vi "IO.vi"() -> ()   [LabVIEW 2010]
panel:
  out "FPGAVersion":i32
  out "HardwareVersion":i32
  out "FirmwareVersion":string
  out "Digital Output 2":bool[](array[boolean])
  out "Digital Output 1":bool[](array[boolean])
  out "Digital Output 0":bool[](array[boolean])
  out "Digital Input 2":bool[](array[boolean])
  out "Digital Input 1":bool[](array[boolean])
  out "Digital Input 0":bool[](array[boolean])
  out "Analog Output 1":dbl
  out "Analog Output 0":dbl
  out "Analog Input 1":dbl
  out "Analog Input 0":dbl
  in  "Analog Output 1 (set)":dbl=-3.25
  in  "Analog Output 0 (set)":dbl=7.0
  in  "Digital Output 2 (set)":i32=255 format="%02x"
  in  "Digital Output 1 (set)":i32=122 format="%02x"
  in  "Digital Output 0 (set)":i32=3 format="%01x"
  in  "Axis Name":string="X"
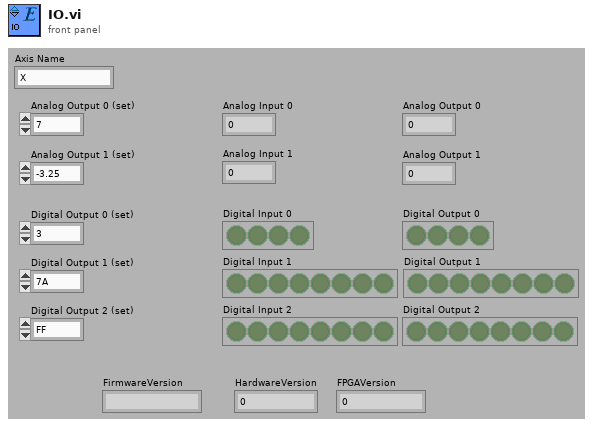
[diagram p1: front panel]
types:
  T1 = typedef "ControllerDiagPacket.ctl" = cluster{"Count":i32, "Packet Time":i64, "Axes":T2[], "error":errorcluster}
  T2 = typedef "AxisDiagPacket.ctl" = cluster{"Axis Name":string, "Acceleration Command":dbl, "Amplifier Temperature":sgl, "Analog Input 0":dbl, "Analog Input 1":dbl, "Analog Output 0":dbl, "Analog Output 1":dbl, "Axis Fault (num)":i32, "Axis Fault (str)":string, "Axis Fault (bits)":cluster{"AmplifierFault":bool, "AmplifierTemperatureFault":bool, "CcwEndOfTravelLimitFault":bool, "CcwSoftwareLimitFault":bool, "CommunicationLostFault":bool, "CwEndOfTravelLimitFault":bool, "CwSoftwareLimitFault":bool, "EmergencyStopFault":bool, "EncoderFault":bool, "ExternalFault":bool, "FeedbackScalingFault":bool, "HallSensorFault":bool, "MarkerSearchFault":bool, "MaxVelocityCommandFault":bool, "MotorTemperatureFault":bool, "None":bool, "OverCurrentFault":bool, "PositionErrorFault":bool, "PositionFeedbackFault":bool, "PowerSupplyFault":bool, "VelocityErrorFault":bool, "VelocityFeedbackFault":bool, "VoltageClampFault":bool}, "Axis Status (num)":i32, "Axis Status (str)":string, "Axis Status (bits)":cluster{"AccelerationPhase":bool, "AutofocusActive":bool, "BrakeOutput":bool, "CalibrationActive":bool, "CalibrationEnabled":bool, "CcwEndOfTravelLimitInput":bool, "CommandShapingFilterDone":bool, "CosineEncoderError":bool, "CurrentClamp":bool, "CwEndOfTravelLimitInput":bool, "DecelerationPhase":bool, "EmergencyStopInput":bool, "Enabled":bool, "GantryMasterActive":bool, "GantryModeActive":bool, "HallAInput":bool, "HallBInput":bool, "HallCInput":bool, "Homed":bool, "HomeLimitInput":bool, "Homing":bool, "InPosition":bool, "InPosition2":bool, "JoystickControl":bool, "MarkerInput":bool, "MasterMotionSuppressed":bool, "MasterSlaveControl":bool, "MotionIsCw":bool, "MoveActive":bool, "None":bool, "PositionCaptureActive":bool, "ServoControl":bool, "SineEncoderError":bool}, "Current Command":sgl, "Current Error":sgl, "Current Feedback":sgl, "Digital Input 0":i32, "Digital Input 1":i32, "Digital Input 2":i32, "Digital Output 0":i32, "Digital Output 1":i32, "Digital Output 2":i32, "Position Feedback Auxiliary":dbl, "Position Command":dbl, "Position Error":dbl, "Position Feedback":dbl, "Program Position Command":dbl, "Program Position Error":dbl, "Program Position Feedback":dbl, "Velocity Command":dbl, "Velocity Error":dbl, "Velocity Feedback":dbl}
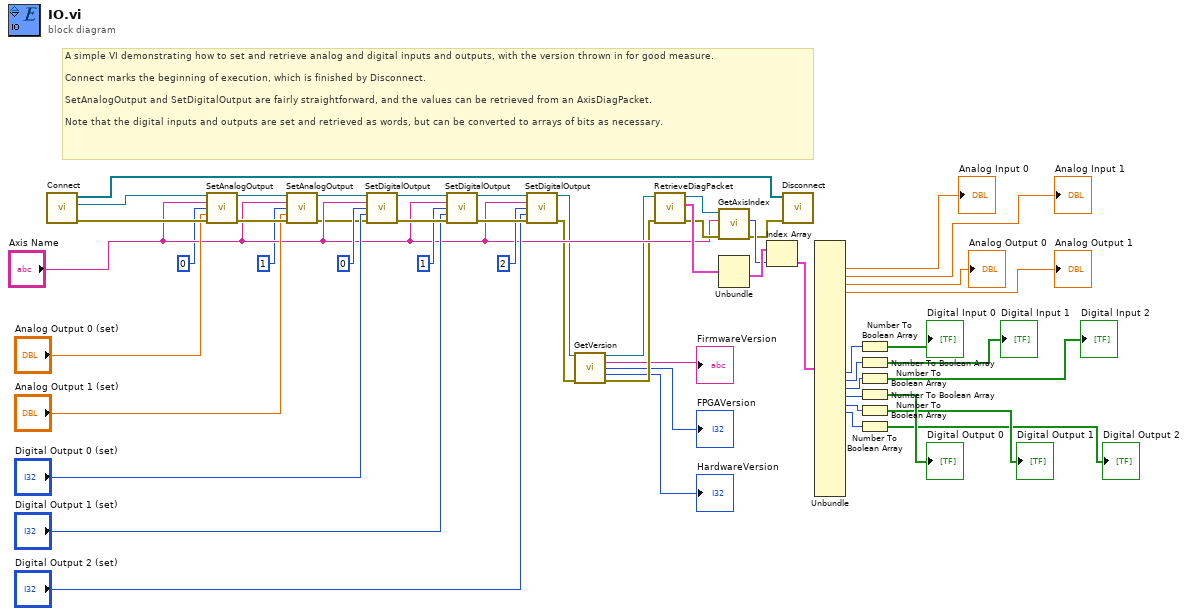
[diagram p0: block diagram]
diagram:
  # "A simple VI demonstrating how to set and retrieve analog and digital inputs and outputs, with the version thrown in for good measure.\n\nConnect marks the beginning of execution, which is finished by Disconnect.\n\nSetAnalogOutput and SetDigitalOutput are fairly straightforward, and the values can be retrieved from an AxisDiagPacket.\n\nNote that the digital inputs and outputs are set and retrieved as words, but can be converted to arrays of bits as necessary."
  n1 = call "Connect.vi"() -> ("error out"=w24:errorcluster, "controller"=w25:refnum<k24>, "controllers"=w7:refnum<k24>[])  [unwired: 9 in]
  n2 = call "SetAnalogOutput.vi"("controller in"=w25, "axis name"="Axis Name", "port"=0 ("Port"), "value"="Analog Output 0 (set)", "error in (no error)"=w24) -> ("controller out"=w23:refnum<k24>, "error out"=w22:errorcluster)  [unwired: 9 in]
  n3 = call "SetAnalogOutput.vi"("controller in"=w23, "axis name"="Axis Name", "port"=1 ("Port"), "value"="Analog Output 1 (set)", "error in (no error)"=w22) -> ("controller out"=w16:refnum<k24>, "error out"=w15:errorcluster)  [unwired: 9 in]
  n4 = call "SetDigitalOutput.vi"("controller in"=w16, "axis name"="Axis Name", "port"=0 ("Port"), "value"="Digital Output 0 (set)", "error in (no error)"=w15) -> ("controller out"=w35:refnum<k24>, "error out"=w33:errorcluster)  [unwired: 9 in]
  n5 = call "SetDigitalOutput.vi"("controller in"=w35, "axis name"="Axis Name", "port"=1 ("Port"), "value"="Digital Output 1 (set)", "error in (no error)"=w33) -> ("controller out"=w34:refnum<k24>, "error out"=w32:errorcluster)  [unwired: 9 in]
  n6 = call "SetDigitalOutput.vi"("controller in"=w34, "axis name"="Axis Name", "port"=2 ("Port"), "value"="Digital Output 2 (set)", "error in (no error)"=w32) -> ("controller out"=w14:refnum<k24>, "error out"=w11:errorcluster)  [unwired: 9 in]
  n7 = call "GetVersion.vi"("controller in"=w14, "error in (no error)"=w11) -> ("controller out"=w13:refnum<k24>, "firmware version"=→"FirmwareVersion":string, "fpga version"=→"FPGAVersion":i32, "hardware version"=→"HardwareVersion":i32, "error out"=w12:errorcluster)  [unwired: 9 in]
  n8 = call "RetrieveDiagPacket.vi"("error in (no error)"=w12, "Controller In"=w13) -> ("error out"=w51:errorcluster, "ControllerDiagPacket"=w52:T1, "Controller Out"=w50:refnum<k24>)  [unwired: 7 in]
  n9 = call "GetAxisIndex.vi"("error in (no error)"=w51, "axis name"="Axis Name", "controller in"=w50) -> ("error out"=w36:errorcluster, "axis index"=w48:i32)  [unwired: 6 in, 1 out]
  n10 = Unbundle(w52) -> ("Axes"=w49:T2[])  [unwired: 3 out]
  n11 = Index Array(array=w49, index=w48) -> (element=w47:T2)
  n12 = call "Disconnect.vi"("error in (no error)"=w36, "controllers"=w7) -> ()  [unwired: 9 in, 1 out]
  n13 = Unbundle(w47) -> ("Analog Input 0"=→"Analog Input 0":dbl, "Analog Input 1"=→"Analog Input 1":dbl, "Analog Output 0"=→"Analog Output 0":dbl, "Analog Output 1"=→"Analog Output 1":dbl, "Digital Input 0"=w1:i32, "Digital Input 1"=w2:i32, "Digital Input 2"=w3:i32, "Digital Output 0"=w4:i32, "Digital Output 1"=w5:i32, "Digital Output 2"=w6:i32)  [unwired: 22 out]
  n14 = Number To Boolean Array(number=w1) -> (Boolean array=→"Digital Input 0":bool[])
  n15 = Number To Boolean Array(number=w2) -> (Boolean array=→"Digital Input 1":bool[])
  n16 = Number To Boolean Array(number=w3) -> (Boolean array=→"Digital Input 2":bool[])
  n17 = Number To Boolean Array(number=w4) -> (Boolean array=→"Digital Output 0":bool[])
  n18 = Number To Boolean Array(number=w5) -> (Boolean array=→"Digital Output 1":bool[])
  n19 = Number To Boolean Array(number=w6) -> (Boolean array=→"Digital Output 2":bool[])
